vi "Create.vi"(10 "Group":refnum<class "Group.lvclass">) -> (3 "GroupValue out":refnum<class "GroupValue.lvclass">)   [LabVIEW 2020, in "Vecto.lvlib" / "GroupValue.lvclass"]
uses:
  GroupValue.lvclass
  Group/Group.lvclass
  GroupValue.lvclass/GroupValue.ctl
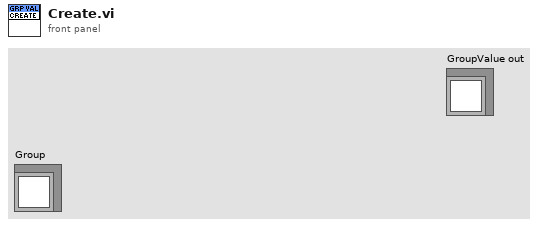
[diagram p1: front panel]
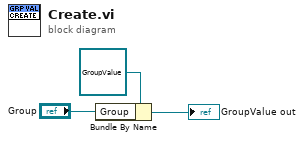
[diagram p0: block diagram]
diagram:
  n1 = Bundle By Name(cluster=refnum<class "GroupValue.lvclass"> refnum ("GroupValue out"), "Group"="Group") -> (→"GroupValue out":refnum<class "GroupValue.lvclass">)
